vi "SendRefillNotification.vi"(11 "Valves IN":u16[](array[ring]) items=["A1", "A2", "A3", "A4", "B1", "B2", "B3", "B4", "B5", "B6", "B7", "B8", "A5", "A6", "A7", "A8"]) -> ()   [LabVIEW 2016]
uses:
  <userlib>/_OpenG.lib/array/array.llb/Index 1D Array Elements (String)__ogtk.vi
  Labjack/ValveGlobals.vi
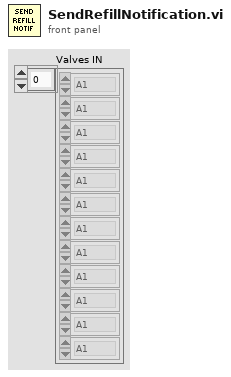
[diagram p1: front panel]
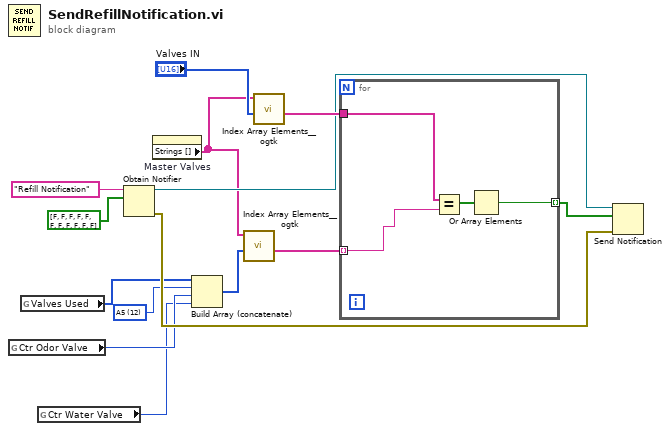
[diagram p0: block diagram]
diagram:
  w5 = u16 12 items=["A1", "A2", "A3", "A4", "B1", "B2", "B3", "B4", "B5", "B6", "B7", "B8", "A5", "A6", "A7", "A8"] ("Master Valves")
  n1 = global read "ValveGlobals.vi" "Ctr Odor Valve"() -> (w4:u16)
  n2 = global read "ValveGlobals.vi" "Valves Used"() -> (w6:u16[])
  n3 = global read "ValveGlobals.vi" "Ctr Water Valve"() -> (w3:u16)
  n4 = Obtain Notifier(name (unnamed)="Refill Notification", notification data type=bool[] [FALSE, FALSE, FALSE, FALSE, FALSE, FALSE, FALSE, FALSE, FALSE, FALSE, FALSE] ("Refill!")) -> (notifier out=w10:refnum<notifier>, error out=w8:errorcluster)  [unwired: 2 in, 1 out]
  n5 = property on="Master Valves" class="Ring (strict)"() -> ("Strings []"=w1:string[])  [unwired: 2 in, 2 out]
  n6 = Build Array (concatenate)(w6, w5, w4, w3) -> (w2:u16[])
  n7 = call-poly <userlib>:"Index Array Elements__ogtk.vi"("indices"=w2, "array"=w1) -> ("elements"=w11:string[])  [unwired: 9 in]
  n8 = call-poly <userlib>:"Index Array Elements__ogtk.vi"("indices"="Valves IN", "array"=w1) -> ("elements"=w12:string[])  [unwired: 9 in]
  n9 = for {
    tunnel: w12 -> [w17]
    tunnel: w11 -> [w18] mode=indexing
    tunnel: [w15] -> w9 mode=indexing
    n10 = Equal?(x=w17, y=w18) -> (x = y?=w16:bool[])
    n11 = Or Array Elements(Boolean array=w16) -> (logical OR=w15:bool)
  }
  n12 = Send Notification(notification=w9, notifier=w10, error in (no error)=w8) -> ()  [unwired: 2 out]
